vi "myRIO_BRig_host_test_main.vi"() -> ()   [LabVIEW 2014]
panel:
  out "subarray":u16[](graph)
  in  "stop":bool
  in  "nTrial_perBlock":u16=5
  in  "nTrial_total":u16=500
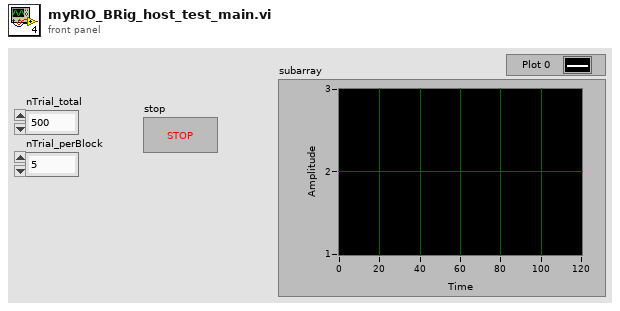
[diagram p1: front panel]
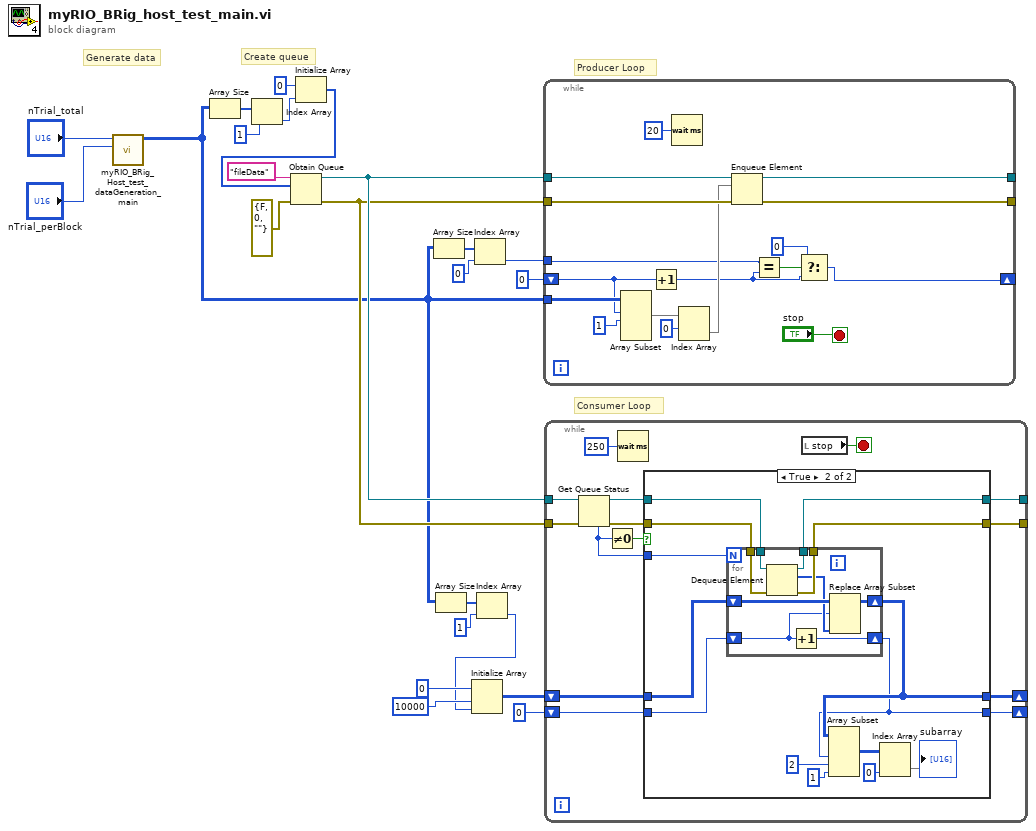
[diagram p0: block diagram]
diagram:
  # "Consumer Loop"
  # "Producer Loop"
  # "Create queue"
  # "Generate data"
  n1 = call "myRIO_BRig_Host_test_dataGeneration_main.vi"("nTrial_perBlock"="nTrial_perBlock", "nTrial_total"="nTrial_total") -> ("output_fileData"=w6:u16[][])  [unwired: 8 in, 1 out]
  n2 = Array Size(array=w6) -> (size(s)=w21:i32[])
  n3 = Index Array(array=w21, index=1) -> (element=w19:i32)
  n4 = Initialize Array(u16 0 ("element"), w19) -> (w17:u16[])
  n5 = Obtain Queue(name (unnamed)="fileData", element data type=w17, error in (no error)=errorcluster {"status"=FALSE, "code"=0, "source"=""}) -> (queue out=w10:refnum<queue>, error out=w9:errorcluster)  [unwired: 2 in, 1 out]
  n6 = Array Size(array=w6) -> (size(s)=w13:i32[])
  n7 = Array Size(array=w6) -> (size(s)=w8:i32[])
  n8 = Index Array(array=w13, index=0) -> (element=w11:i32)
  n9 = Index Array(array=w8, index=1) -> (element=w3:i32)
  n10 = Initialize Array(u16 0 ("element"), 10000 ("dimension size"), w3) -> (w2:u16[][])
  n11 = while {
    tunnel: w6 -> [w39]
    shift-right: [w24] -> _
    shift-left: 0 ("index") -> [w38]
    tunnel: w10 -> [w37]
    tunnel: w9 -> [w36]
    tunnel: w11 -> [w29]
    tunnel: [w32] -> _
    tunnel: [w31] -> _
    stop <- "stop" stop-if-true
    n12 = Array Subset(array=w39, index (row)=w38, length (row)=1 ("length")) -> (w34:u16[][])  [unwired: 2 in]
    n13 = Increment(x=w38) -> (x+1=w27:i32)
    n14 = Wait (ms)(milliseconds to wait=u32 20) -> ()  [unwired: 1 out]
    n15 = Index Array(array=w34, index (row)=0) -> (element=w33:u16[])  [unwired: 1 in]
    n16 = Enqueue Element(queue=w37, element=w33, error in (no error)=w36) -> (queue out=w31:refnum<queue>, error out=w32:errorcluster)  [unwired: 1 in, 1 out]
    n17 = Equal?(x=w29, y=w27) -> (x = y?=w28:bool)
    n18 = Select(t=0, s=w28, f=w27) -> (s? t:f=w24:i32)
  }
  n19 = while {
    tunnel: w10 -> [w51]
    tunnel: w9 -> [w50]
    tunnel: [w53] -> _
    tunnel: [w52] -> _
    shift-right: [w43] -> _
    shift-left: w2 -> [w44]
    shift-right: [w41] -> _
    shift-left: 0 ("element") -> [w42]
    stop <- w47 stop-if-true
    n20 = Get Queue Status(queue=w51, error in (no error)=w50) -> (queue out=w49:refnum<queue>, error out=w48:errorcluster, # elements in queue=w45:i32)  [unwired: 1 in, 5 out]
    n21 = Not Equal To 0?(x=w45) -> (x != 0?=w46:bool)
    n22 = Wait (ms)(milliseconds to wait=u32 250) -> ()  [unwired: 1 out]
    n23 = case shown="True" w46 {
      tunnel: [w57 w69] -> w53
      tunnel: [w58 w70] -> w52
      tunnel: w49 -> [w58 w72]
      tunnel: w48 -> [w57 w71]
      tunnel: w45 -> [_ w68]
      tunnel: w44 -> [w56 w67]
      tunnel: [w56 w65] -> w43
      tunnel: w42 -> [w55 w66]
      tunnel: [w55 w64] -> w41
      frame False {
      }
      frame True {
        n24 = for {
          N: w68 -> [_]
          tunnel: w72 -> [w81]
          tunnel: w71 -> [w80]
          tunnel: [w79] -> w70
          tunnel: [w78] -> w69
          shift-right: [w77] -> w65
          shift-left: w67 -> [w76]
          shift-right: [w74] -> w64
          shift-left: w66 -> [w73]
          n25 = Dequeue Element(queue=w81, error in (no error)=w80) -> (queue out=w79:refnum<queue>, element=w75:u16[], error out=w78:errorcluster)  [unwired: 1 in, 1 out]
          n26 = Increment(x=w73) -> (x+1=w74:i32)
          n27 = Replace Array Subset(array=w76, new element=w75, index (row)=w73) -> (w77:u16[][])  [unwired: 1 in]
        }
        n28 = Array Subset(array=w65, length (row)=w64, index (col)=2 ("index"), length (col)=1 ("length")) -> (w61:u16[][])  [unwired: 1 in]
        n29 = Index Array(array=w61, index (col)=0 ("disabled index (col)")) -> (element=→"subarray":u16[])  [unwired: 1 in]
      }
    }
    n30 = local read "stop"() -> (w47:bool)
  }
